vi "BARCODE_SEARCH.vi"(8 "error in":errorcluster, 9 "BARCODE_TABLE":string[][](table), 11 "BARCODE_TO_SEARCH":string) -> (0 "error out":errorcluster, 1 "ARTICLE name":string, 2 "FOUND_ROW":string[](array[string]), 3 "BARCODE_FOUND":bool, 4 "description NAME":string, 5 "CHL":T1)   [LabVIEW 2017]
panel:
  out "CHL 3":T2
  out "CHL 2":T3
  out "CHL 1":T4
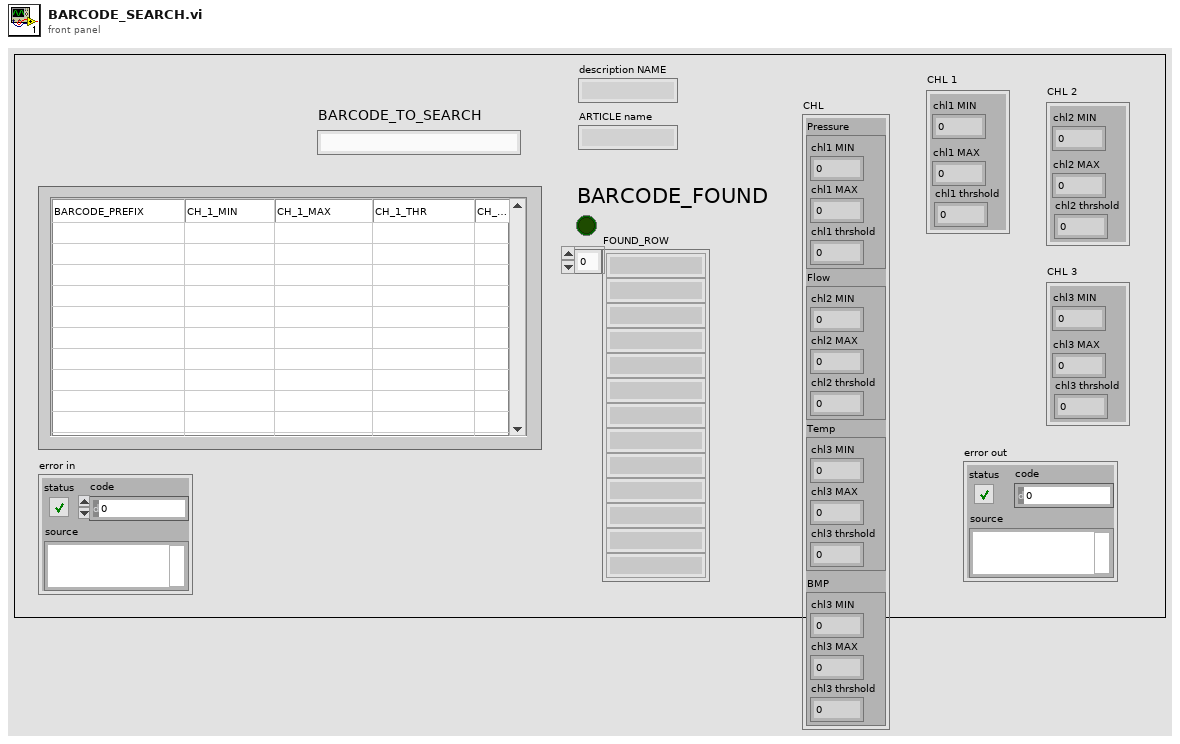
[diagram p1: front panel]
types:
  T1 = cluster{"Pressure":cluster{"chl1 MIN":dbl, "chl1 MAX":dbl, "chl1 thrshold":dbl}, "Flow":cluster{"chl2 MIN":dbl, "chl2 MAX":dbl, "chl2 thrshold":dbl}, "Temp":cluster{"chl3 MIN":dbl, "chl3 MAX":dbl, "chl3 thrshold":dbl}, "BMP":cluster{"chl3 MIN":dbl, "chl3 MAX":dbl, "chl3 thrshold":dbl}}
  T2 = cluster{"chl3 MIN":dbl, "chl3 MAX":dbl, "chl3 thrshold":dbl}
  T3 = cluster{"chl2 MIN":dbl, "chl2 MAX":dbl, "chl2 thrshold":dbl}
  T4 = cluster{"chl1 MIN":dbl, "chl1 MAX":dbl, "chl1 thrshold":dbl}
  T5 = cluster{"Pressure":cluster{"chl1 MIN":dbl, "chl1 MAX":dbl, "chl1 thrshold":dbl}, "Flow":cluster{"chl2 MIN":dbl, "chl2 MAX":dbl, "chl2 thrshold":dbl}, "Temp":cluster{"chl3 MIN":dbl, "chl3 MAX":dbl, "chl3 thrshold":dbl}, "BMP":cluster{"chl2 MIN":dbl, "chl2 MAX":dbl, "chl2 thrshold":dbl}}
  T6 = cluster{"element":dbl, "element":dbl, "element":dbl}
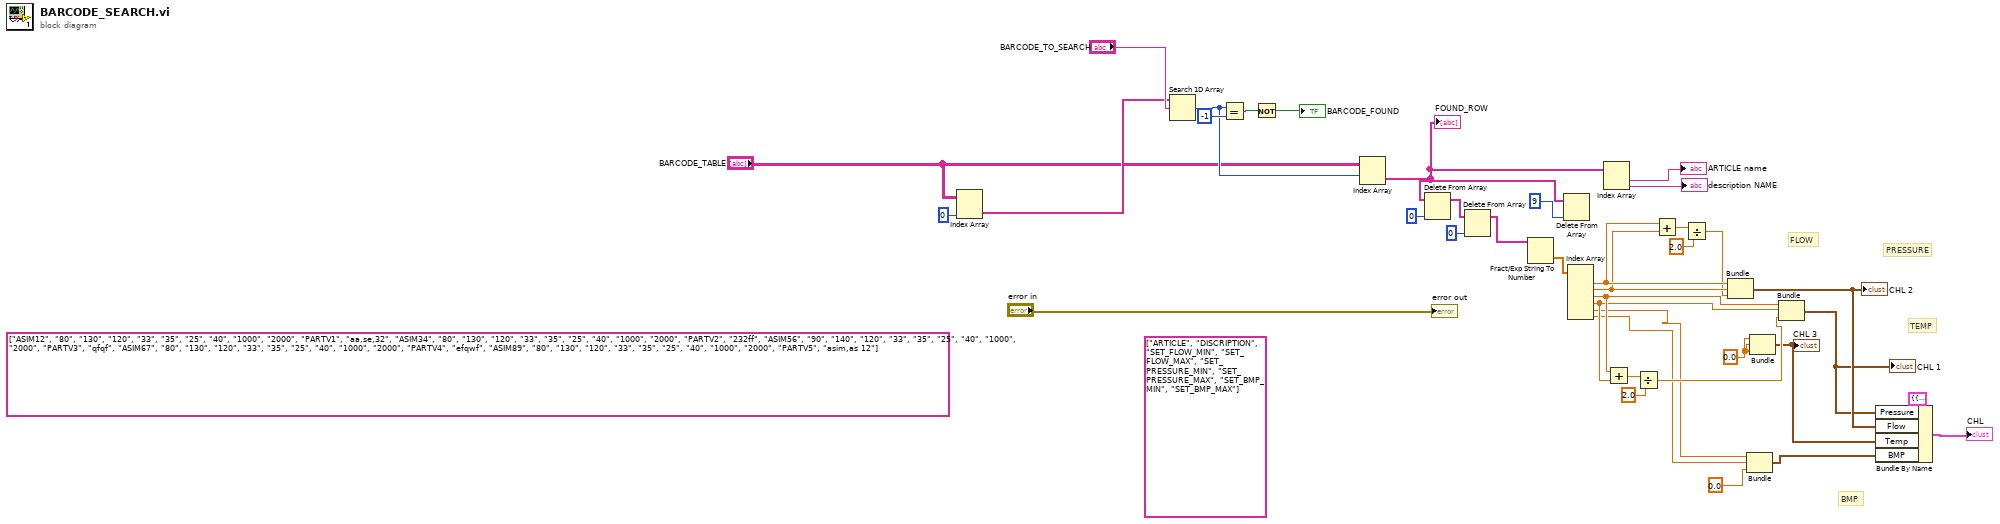
[diagram p0: block diagram]
diagram:
  (unwired) string[] ["ARTICLE", "DISCRIPTION", "SET_FLOW_MIN", "SET_FLOW_MAX", "SET_PRESSURE_MIN", "SET_PRESSURE_MAX", "SET_BMP_MIN", "SET_BMP_MAX"] ("columns 2")
  (unwired) string[][] [["ASIM12", "80", "130", "120", "33", "35", "25", "40", "1000", "2000", "PARTV1", "aa,se,32"], ["ASIM34", "80", "130", "120", "33", "35", "25", "40", "1000", "2000", "PARTV2", "232ff"], ["ASIM56", "90", "140", "120", "33", "35", "25", "40", "1000", "2000", "PARTV3", "qfqf"], ["ASIM67", "80", "130", "120", "33", "35", "25", "40", "1000", "2000", "PARTV4", "efqwf"], ["ASIM89", "80", "130", "120", "33", "35", "25", "40", "1000", "2000", "PARTV5", "asim,as 12"]] ("table")
  w2 = 0.0 ("element")
  # "BMP"
  # "TEMP"
  # "PRESSURE"
  # "FLOW"
  n1 = Index Array(array="BARCODE_TABLE", index (col)=0 ("disabled index (col)")) -> (element=w29:string[])  [unwired: 1 in]
  n2 = Search 1D Array(1D array=w29, element="BARCODE_TO_SEARCH") -> (index of element=w34:i32)  [unwired: 1 in]
  n3 = Equal?(x=w34, y=-1) -> (x = y?=w37:bool)
  n4 = Not(x=w37) -> (.not. x?=→"BARCODE_FOUND":bool)
  n5 = Index Array(array="BARCODE_TABLE", index (row)=w34) -> (element=w16:string[])  [unwired: 1 in]
  "FOUND_ROW" <- w16
  n6 = Delete From Array(array=w16, index=0) -> (array with subset deleted=w17:string[])  [unwired: 1 in, 1 out]
  n7 = Delete From Array(array=w17, index=0) -> (array with subset deleted=w15:string[])  [unwired: 1 in, 1 out]
  n8 = Fract/Exp String To Number(string=w15) -> (number=w31:dbl[])  [unwired: 3 in, 1 out]
  n9 = Delete From Array(array=w16, index=9) -> ()  [unwired: 1 in, 2 out]
  n10 = Index Array(array=w31) -> (element #1=w14:dbl, element #2=w13:dbl, element #3=w8:dbl, element #4=w7:dbl, element #5=w4:dbl, element #6=w3:dbl)  [unwired: 6 in]
  n11 = Index Array(array=w16) -> (element #1=→"ARTICLE name":string, element #2=→"description NAME":string)  [unwired: 2 in]
  n12 = Add(x=w8, y=w7) -> (x+y=w9:dbl)
  n13 = Divide(x=w9, y=2.0) -> (x/y=w6:dbl)
  n14 = Add(x=w14, y=w13) -> (x+y=w20:dbl)
  n15 = Divide(x=w20, y=2.0) -> (x/y=w12:dbl)
  n16 = Bundle(w14, w13, w12) -> (w11:cluster{dbl, dbl, dbl})  [unwired: 1 in]
  "CHL 2" <- w11
  n17 = Bundle(w4, w3, "element"=0.0) -> (w23:cluster{dbl, dbl, "element":dbl})  [unwired: 1 in]
  n18 = Bundle("element"=w2, "element"=w2, "element"=w2) -> (w1:T6)  [unwired: 1 in]
  "CHL 3" <- w1
  n19 = Bundle(w8, w7, w6) -> (w5:cluster{dbl, dbl, dbl})  [unwired: 1 in]
  "CHL 1" <- w5
  n20 = Bundle By Name(cluster=T5 {"Pressure"={"chl1 MIN"=110.0, "chl1 MAX"=130.0, "chl1 thrshold"=120.0}, "Flow"={"chl2 MIN"=33.0, "chl2 MAX"=35.0, "chl2 thrshold"=25.0}, "Temp"={"chl3 MIN"=20.0, "chl3 MAX"=30.0, "chl3 thrshold"=34.0}, "BMP"={"chl2 MIN"=33.0, "chl2 MAX"=35.0, "chl2 thrshold"=25.0}}, "Pressure"=w5, "Flow"=w11, "Temp"=w1, "BMP"=w23) -> (→"CHL":T5)
  "error out" <- "error in"
